vi "Inject Attribute List.vi"(6 "Attributes Ref":refnum<data-value>, 8 "error in (no error)":errorcluster, 11 "Start Pre-Soak in":refnum<class "Start Air Dry.lvclass">) -> (0 "error out":errorcluster, 3 "Start Pre-Soak out":refnum<class "Start Air Dry.lvclass">)   [LabVIEW 2019, in "Start Air Dry.lvclass"]
uses:
  <vilib>/gpm_packages/@cs/Car-wash/Source/Process Steps/Start Air Dry/Start Air Dry.lvclass
  <vilib>/gpm_packages/@cs/lookup-table/Source/LookupTable/LookupTable.lvclass
  <vilib>/gpm_packages/@cs/lookup-table/Source/LookupTable/LookupTable.lvclass/LookupTable.ctl
  <vilib>/gpm_packages/@cs/Car-wash/Source/Process Steps/Start Air Dry/Start Air Dry.lvclass/Start Air Dry.ctl
  16f4659b-a4c2-423a-a5d5-b8c487490dd7.vi
  <vilib>/gpm_packages/@cs/lookup-table/Source/LookupTable/Read Table Reference.vi
  16f4659b-a4c2-423a-a5d5-b8c487490dd7.vi/0582fc7e-e07f-432c-9f5f-3805ebeb80a2.vi
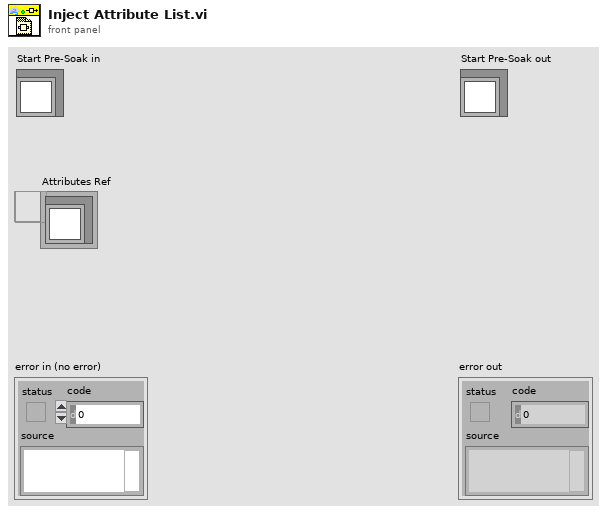
[diagram p1: front panel]
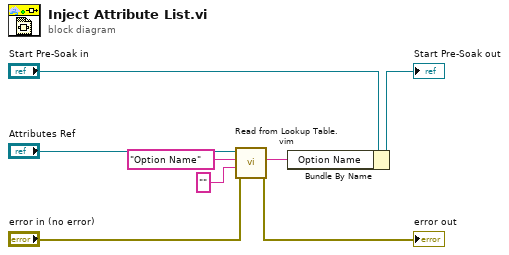
[diagram p0: block diagram]
diagram:
  n1 = call "Read from Lookup Table.vim"("error in (no error)"="error in (no error)", "Type"="", "Item Name"="Option Name", "LookupTable Reference"="Attributes Ref") -> ("error out"=→"error out":errorcluster, "Value"=w3:string)  [unwired: 4 in, 2 out]
  n2 = Bundle By Name(cluster="Start Pre-Soak in", "Option Name"=w3) -> (→"Start Pre-Soak out":refnum<class "Start Air Dry.lvclass">)
